vi "4.7.1.vi"() -> ()   [LabVIEW 2018]
panel:
  out "c":dbl
  in  "연산":enum16{"더하기", "빼기", "곱하기", "나누기"}(ring)
  in  "b":dbl
  in  "a":dbl
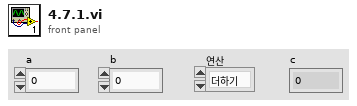
[diagram p1: front panel]
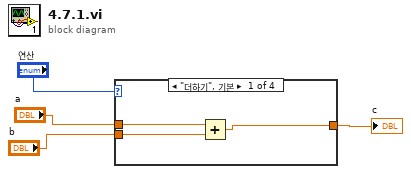
[diagram p0: block diagram]
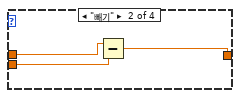
[diagram p2: hidden frame]
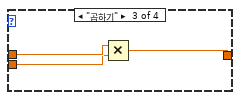
[diagram p3: hidden frame]
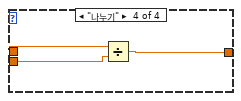
[diagram p4: hidden frame]
diagram:
  n1 = case shown="\"더하기\", 기본" "연산" {
    tunnel: "a" -> [w7 w10 w13 w16]
    tunnel: "b" -> [w6 w9 w12 w15]
    tunnel: [w5 w8 w11 w14] -> w1
    frame "더하기", Default {
      n2 = Add(x=w7, y=w6) -> (x+y=w5:dbl)
    }
    frame "빼기" {
      n3 = Subtract(x=w10, y=w9) -> (x-y=w8:dbl)
    }
    frame "곱하기" {
      n4 = Multiply(x=w13, y=w12) -> (x*y=w11:dbl)
    }
    frame "나누기" {
      n5 = Divide(x=w16, y=w15) -> (x/y=w14:dbl)
    }
  }
  "c" <- w1
